vi "MGI 2D Target 3D Camera.vi"(8 "error in (no error)":errorcluster, 10 "Pane Coordinates":cluster{"X":i32, "Y":i32}, 11 "SceneGraphDisplay in":refnum<vi>) -> (0 "error out":errorcluster, 3 "SceneGraphDisplay out":refnum<vi>)   [LabVIEW 2020]
doc: "Aim the 3D camera at a target specified in pane coordinates (same as Mouse Down event) while maintaining orientation and zoom. Z-up orientation is assumed.\n\nAuthored by David A. Moore\nsupport@mooregoodideas.com\nwww.mooregoodideas.com\n\nCopyright (c) 2012, Moore Good Ideas, Inc.\n\nAll rights reserved.\n\nRedistribution and use in source and binary forms, with or without modification, are permitted provided that the following conditions are met:\n\n * Redistributions of source code must retain the above copyright notice, this list of conditions and the following disclaimer.\n * Redistributions in binary form must reproduce the above copyright notice, this list of conditions and the following disclaimer in the documentation and/or other materials provided with the distribution.\n * Neither the name of Moore Good Ideas, Inc. nor the names of its contributors may be used to endorse or promote products derived from this software without specific prior written permission.\n\nTHIS SOFTWARE IS PROVIDED BY THE COPYRIGHT HOLDERS AND CONTRIBUTORS \"AS IS\" AND ANY EXPRESS OR IMPLIED WARRANTIES, INCLUDING, BUT NOT LIMITED TO, THE IMPLIED WARRANTIES OF MERCHANTABILITY AND FITNESS FOR A PARTICULAR PURPOSE ARE DISCLAIMED. IN NO EVENT SHALL THE COPYRIGHT OWNER OR CONTRIBUTORS BE LIABLE FOR ANY DIRECT, INDIRECT, INCIDENTAL, SPECIAL, EXEMPLARY, OR CONSEQUENTIAL DAMAGES (INCLUDING, BUT NOT LIMITED TO, PROCUREMENT OF SUBSTITUTE GOODS OR SERVICES; LOSS OF USE, DATA, OR PROFITS; OR BUSINESS INTERRUPTION) HOWEVER CAUSED AND ON ANY THEORY OF LIABILITY, WHETHER IN CONTRACT, STRICT LIABILITY, OR TORT (INCLUDING NEGLIGENCE OR OTHERWISE) ARISING IN ANY WAY OUT OF THE USE OF THIS SOFTWARE, EVEN IF ADVISED OF THE POSSIBILITY OF SUCH DAMAGE."
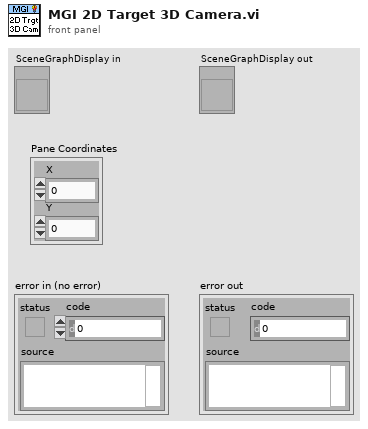
[diagram p1: front panel]
types:
  T1 = typedef "LVPositionTypeDef.ctl" = cluster{"Left":i32, "Top":i32}
  T2 = typedef "LV3DPointTypeDef.ctl" = cluster{"X":sgl, "Y":sgl, "Z":sgl}
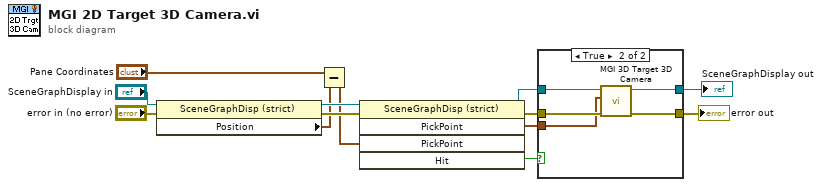
[diagram p0: block diagram]
diagram:
  n1 = property on="Property Node" class="SceneGraphDisp (strict)"(reference="SceneGraphDisplay in", error in="error in (no error)") -> (reference out=w8:refnum<vi>, error out=w7:errorcluster, "Position"=w4:T1)
  n2 = Subtract(x="Pane Coordinates", y=w4) -> (x-y=w3:T1)
  n3 = invoke class="SceneGraphDisp (strict)" method="PickPoint"(reference=w8, error in=w7, "PickPoint"=w3) -> (reference out=w6:refnum<vi>, error out=w5:errorcluster, "PickPoint"=w1:T2, "Hit"=w2:bool)  [unwired: 2 in, 1 out]
  n4 = case shown="True" w2 {
    tunnel: [w14 w16] -> w13
    tunnel: [w15 w17] -> w10
    tunnel: w6 -> [w14 w20]
    tunnel: w5 -> [w15 w19]
    tunnel: w1 -> [_ w18]
    frame False {
    }
    frame True {
      n5 = call <userlib>:"MGI 3D Target 3D Camera.vi"("error in (no error)"=w19, "3D Target"=w18, "SceneGraphDisplay in"=w20) -> ("error out"=w17:errorcluster, "SceneGraphDisplay out"=w16:refnum<vi>)  [unwired: 7 out]
    }
  }
  "SceneGraphDisplay out" <- w13
  "error out" <- w10
